vi "ResetPanelValues.vi"(4 "Abort":refnum<vi>, 5 "Fire Experiment":refnum<vi>, 6 "Discard shot data":refnum<vi>, 7 "Save shot data":refnum<vi>) -> ()   [LabVIEW 2015]
doc: "Resets certain front panel button values to the default (program-initialized) values."
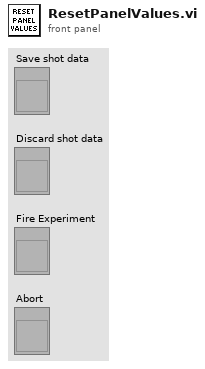
[diagram p1: front panel]
types:
  T1 = enum8{"Enabled", "Disabled", "Disabled and Grayed Out"}
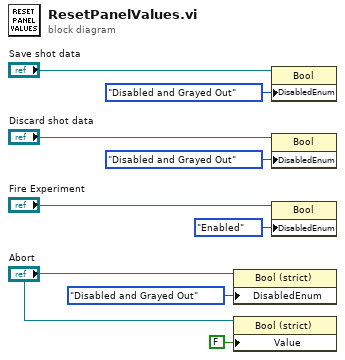
[diagram p0: block diagram]
diagram:
  n1 = property class="Bool (strict)"(reference="Abort", "DisabledEnum"=T1."Disabled and Grayed Out" ("Disabled")) -> ()  [unwired: 1 in, 2 out]
  n2 = property class="Bool (strict)"(reference="Abort", "Value"=FALSE) -> ()  [unwired: 1 in, 2 out]
  n3 = property class="Bool"(reference="Save shot data", "DisabledEnum"=T1."Disabled and Grayed Out" ("Disabled")) -> ()  [unwired: 1 in, 2 out]
  n4 = property class="Bool"(reference="Discard shot data", "DisabledEnum"=T1."Disabled and Grayed Out" ("Disabled")) -> ()  [unwired: 1 in, 2 out]
  n5 = property class="Bool"(reference="Fire Experiment", "DisabledEnum"=T1."Enabled" ("Disabled")) -> ()  [unwired: 1 in, 2 out]
